vi "DataAcquisition.vi"(11 "element":T1) -> (3 "Data":dbl[](array[numeric])=[1.25, 2.5, 3.7, 4.9])   [LabVIEW 2022 SP3]
uses:
  <vilib>/DAQmx/read.llb/DAQmx Read (Analog 1D DBL NChan 1Samp).vi
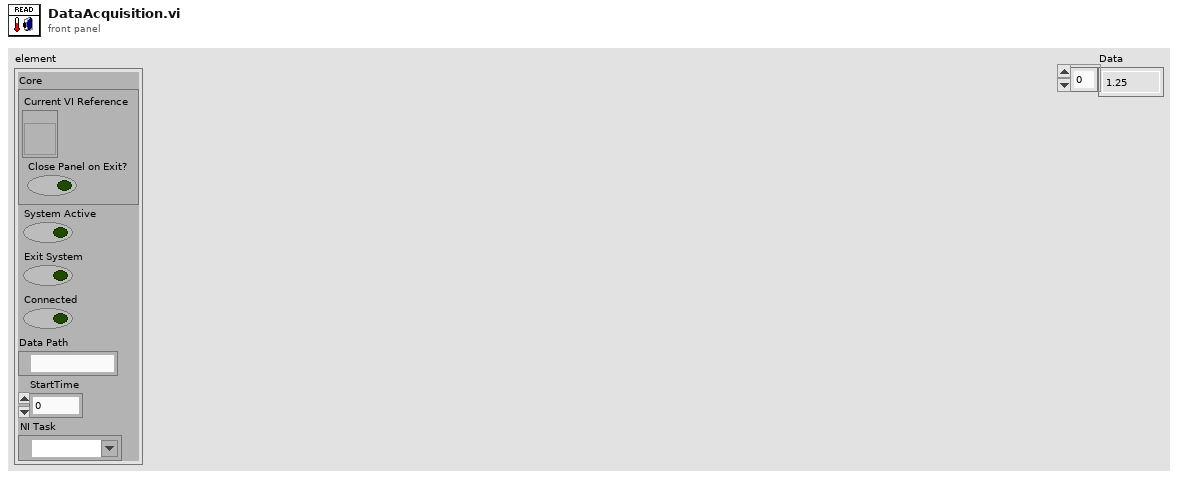
[diagram p1: front panel]
types:
  T1 = cluster{"Core":cluster{"Current VI Reference":refnum<vi>, "Close Panel on Exit?":bool}, "System Active":bool, "Exit System":bool, "Connected":bool, "Data Path":path, "StartTime":u32, "NI Task":refnum<k21>}
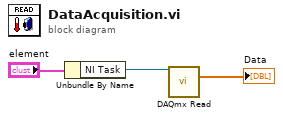
[diagram p0: block diagram]
diagram:
  n1 = Unbundle By Name("element") -> ("NI Task"=w2:refnum<k21>)
  n2 = call-poly <vilib>:"DAQmx Read.vi"("task/channels in"=w2) -> ("data"=→"Data":dbl[])  [unwired: 12 in, 2 out]
